vi "Calculate Mean, Min, Max Values.vi"(11 "Ganged Measurement":dbl[](array[numeric])) -> (1 "Min value":dbl, 2 "Max value":dbl, 3 "Mean value":dbl)   [LabVIEW 2021]
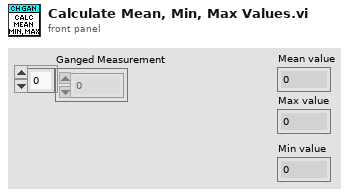
[diagram p1: front panel]
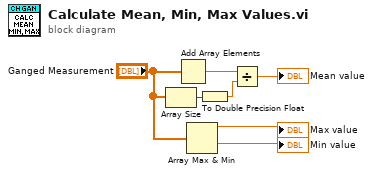
[diagram p0: block diagram]
diagram:
  n1 = Array Size(array="Ganged Measurement") -> (size(s)=w7:i32)
  n2 = Add Array Elements(numeric array="Ganged Measurement") -> (sum=w6:dbl)
  n3 = Array Max & Min(array="Ganged Measurement") -> (max value=→"Max value":dbl, min value=→"Min value":dbl)  [unwired: 2 out]
  n4 = To Double Precision Float(number=w7) -> (double precision float=w1:dbl)
  n5 = Divide(x=w6, y=w1) -> (x/y=→"Mean value":dbl)
